vi "Clear Encoder Data.vi"(0 "reference in":refnum<class "NeedleValve.lvclass">, 11 "error in (no error)":errorcluster) -> (4 "reference out":refnum<class "NeedleValve.lvclass">, 15 "error out":errorcluster)   [LabVIEW 2019, in "NeedleValve.lvclass"]
uses:
  NeedleValve.lvclass
  NeedleValve.lvclass/NeedleValve.ctl
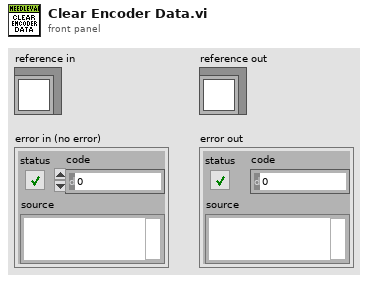
[diagram p1: front panel]
types:
  T1 = typedef "Needle Valve Data.ctl" = cluster{"Engine State":T2, "StateValveModbus":T3, "Alarms":T4, "RAW":i32, "Angele":dbl, "Step":i32, "Encoder":i32, "Kinematic":T5, "Limits":T6, "EncoderMax":i32, "Counter Max Dont Update":i32, "EncoderMin":i32, "Counter Min Dont Update":i32, "Prepere Counter":i32, "STEP INIT":i32, "offset - Angel":dbl}
  T2 = typedef "MB_ENGINE.lvclass/Engine State.ctl" = u16
  T3 = typedef "Needle Valve State.ctl" = enum16{"STOPED", "CLOSED", "OPENED", "OPENING", "CLOSING", "FULL_CLOSE", "PREP_OPEN"}
  T4 = typedef "MB_ENGINE.lvclass/Engine Alarms.ctl" = cluster{"OL":bool, "TF":bool, "STL":bool, "OCP":bool, "CPUV":bool, "UVLO":bool, "SPI_ERROR":bool, "Fault":bool, "OL 2":bool, "TF 2":bool, "STL 2":bool, "OCP 2":bool, "CPUV 2":bool, "UVLO 2":bool, "reserved":bool, "InitDone":bool}
  T5 = typedef "MB_ENGINE.lvclass/Settings.ctl" = cluster{"ACC Steps Per Sec^2":u16, "DEC Steps Per Sec^2":u16, "Min Velosity Step Per Sec":u16, "Max Velosity Step Per Sec":u16, "MicroStep":u16}
  T6 = typedef "MB_ENGINE.lvclass/Limits Status.ctl" = cluster{"Fault 2 Switch":bool, "Fault 1 Switch":bool, "Center(Home)":bool, "Lower Limit":bool, "Upper Limit":bool}
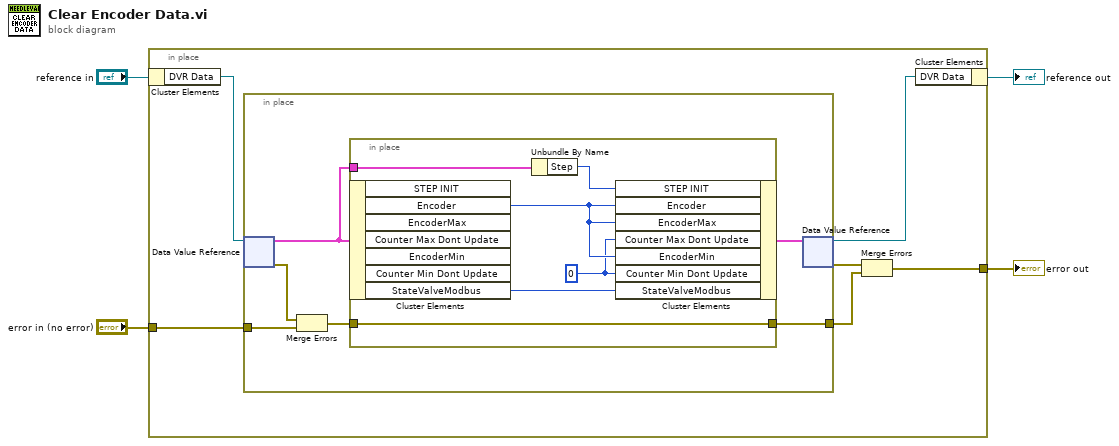
[diagram p0: block diagram]
diagram:
  n1 = in-place {
    in-place-border: "error in (no error)" -> [w10]
    in-place-border: [w6] -> w3
    n2 = in-place-cluster #1("reference in") -> ("DVR Data"=w8:refnum<data-value>)
    n3 = in-place {
      in-place-border: w10 -> [w16]
      in-place-border: [w15] -> w9
      n4 = in-place-dvr #2(w8) -> (w14:T1, w11:errorcluster)
      n5 = Merge Errors(w11, w16) -> (w12:errorcluster)
      n6 = in-place {
        in-place-border: w14 -> [w17]
        in-place-border: w12 -> [w21]
        in-place-border: [w21] -> w15
        w19 = 0 ("Counter Max Dont Update")
        n7 = in-place-cluster #3(w14) -> ("Encoder"=w20:i32, "StateValveModbus"=w22:T3)  [unwired: 5 out]
        n8 = Unbundle By Name(w17) -> ("Step"=w18:i32)
        n9 = in-place-cluster #3("STEP INIT"=w18, "Encoder"=w20, "EncoderMax"=w20, "Counter Max Dont Update"=w19, "EncoderMin"=w20, "Counter Min Dont Update"=w19, "StateValveModbus"=w22) -> (w13:T1)
      }
      n10 = in-place-dvr #2(w13) -> (w7:refnum<data-value>, w5:errorcluster)
    }
    n11 = Merge Errors(w5, w9) -> (w6:errorcluster)
    n12 = in-place-cluster #1("DVR Data"=w7) -> (→"reference out":refnum<class "NeedleValve.lvclass">)
  }
  "error out" <- w3
